vi "Helmholtz2D_FEM_Delaunay_Combine Edge.vi"(10 "New Edges":i32[][](array[numeric]), 11 "Edges in":i32[][](array[numeric])) -> (3 "Edges Out":i32[][](array[numeric]))   [LabVIEW 2020, in "NI_PDE.lvlib"]
uses:
  <vilib>/gmath/NI_PDE.lvlib
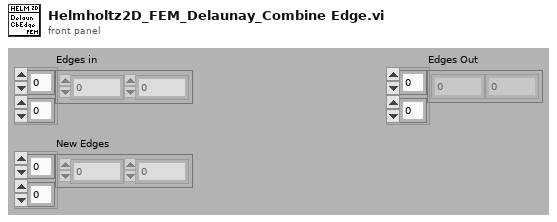
[diagram p1: front panel]
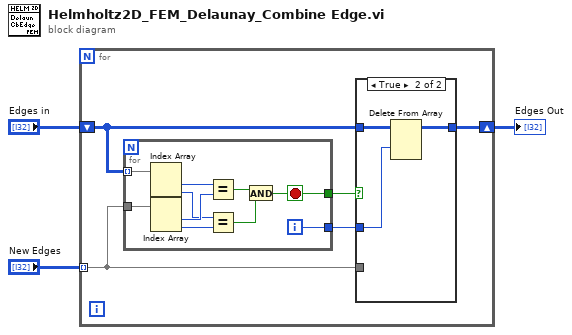
[diagram p0: block diagram]
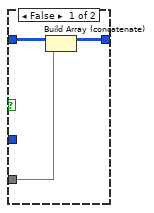
[diagram p2: hidden frame]
diagram:
  n1 = for {
    tunnel: "New Edges" -> [w7] mode=indexing
    shift-right: [w6] -> w3
    shift-left: "Edges in" -> [w8]
    n2 = for {
      tunnel: w8 -> [w23] mode=indexing
      tunnel: w7 -> [w22]
      tunnel: [w15] -> w5
      tunnel: [w24] -> w4
      i -> [w24]
      stop <- w15 stop-if-true
      n3 = Index Array(array=w23) -> (element #1=w21:i32, element #2=w19:i32)  [unwired: 2 in]
      n4 = Index Array(array=w22) -> (element #1=w20:i32, element #2=w18:i32)  [unwired: 2 in]
      n5 = Equal?(x=w21, y=w20) -> (x = y?=w16:bool)
      n6 = Equal?(x=w19, y=w18) -> (x = y?=w17:bool)
      n7 = And(x=w16, y=w17) -> (x .and. y?=w15:bool)
    }
    n8 = case shown="True" w5 {
      tunnel: w8 -> [w11 w14]
      tunnel: w7 -> [w9 _]
      tunnel: [w10 w13] -> w6
      tunnel: w4 -> [_ w12]
      frame False {
        n9 = Build Array (concatenate)(w11, w9) -> (w10:i32[][])
      }
      frame True {
        n10 = Delete From Array(array=w14, index (row)=w12) -> (array with subset deleted=w13:i32[][])  [unwired: 2 in, 1 out]
      }
    }
  }
  "Edges Out" <- w3
